vi "Send signal mode.vi"() -> ()   [LabVIEW 2020]
uses:
  <vilib>/xnet/xnet.llb/XNET Write (Signal Single-point).vi
  <vilib>/xnet/xnet.llb/XNET Create Session (Signal Output Single-point).vi
panel:
  out "校验成功":bool=TRUE
  in  "Close":bool
  in  "CAN1_interface":refnum<k21>="CAN1"
  in  "CAN1":refnum<k21>[](array[refnum])=["Vehicle_speed\nSA2HG", "VehicleSpeed_Status\nSA2HG", "ESP1_MSG_Counter\nSA2HG", "ESP1_Checksum\nSA2HG"]
  in  "CAN1_Write":bool
  in  "CAN1_commd":dbl[](array[numeric])=[0.0, 0.0, 0.0, 0.0] caption="data"
  in  "CAN2_Stop":bool
  in  "CAN1_Stop":bool
  in  "CAN2_Write":bool
  in  "CAN2_commd":dbl[](array[numeric])=[0.0, 0.0, 0.0, 0.0, 0.0] caption="data"
  in  "CAN_Interface":refnum<k21>="CAN1"
  in  "CAN2":refnum<k21>[](array[refnum])=["READY\nSA2HG"]
  # "发送车速信号，时间间隔20ms"
  # "发送Ready信号，时间间隔为100ms"
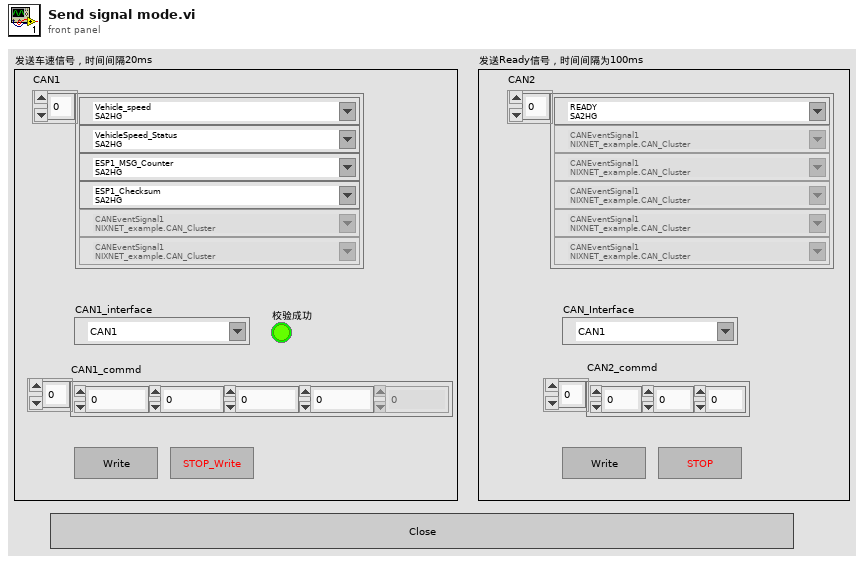
[diagram p1: front panel]
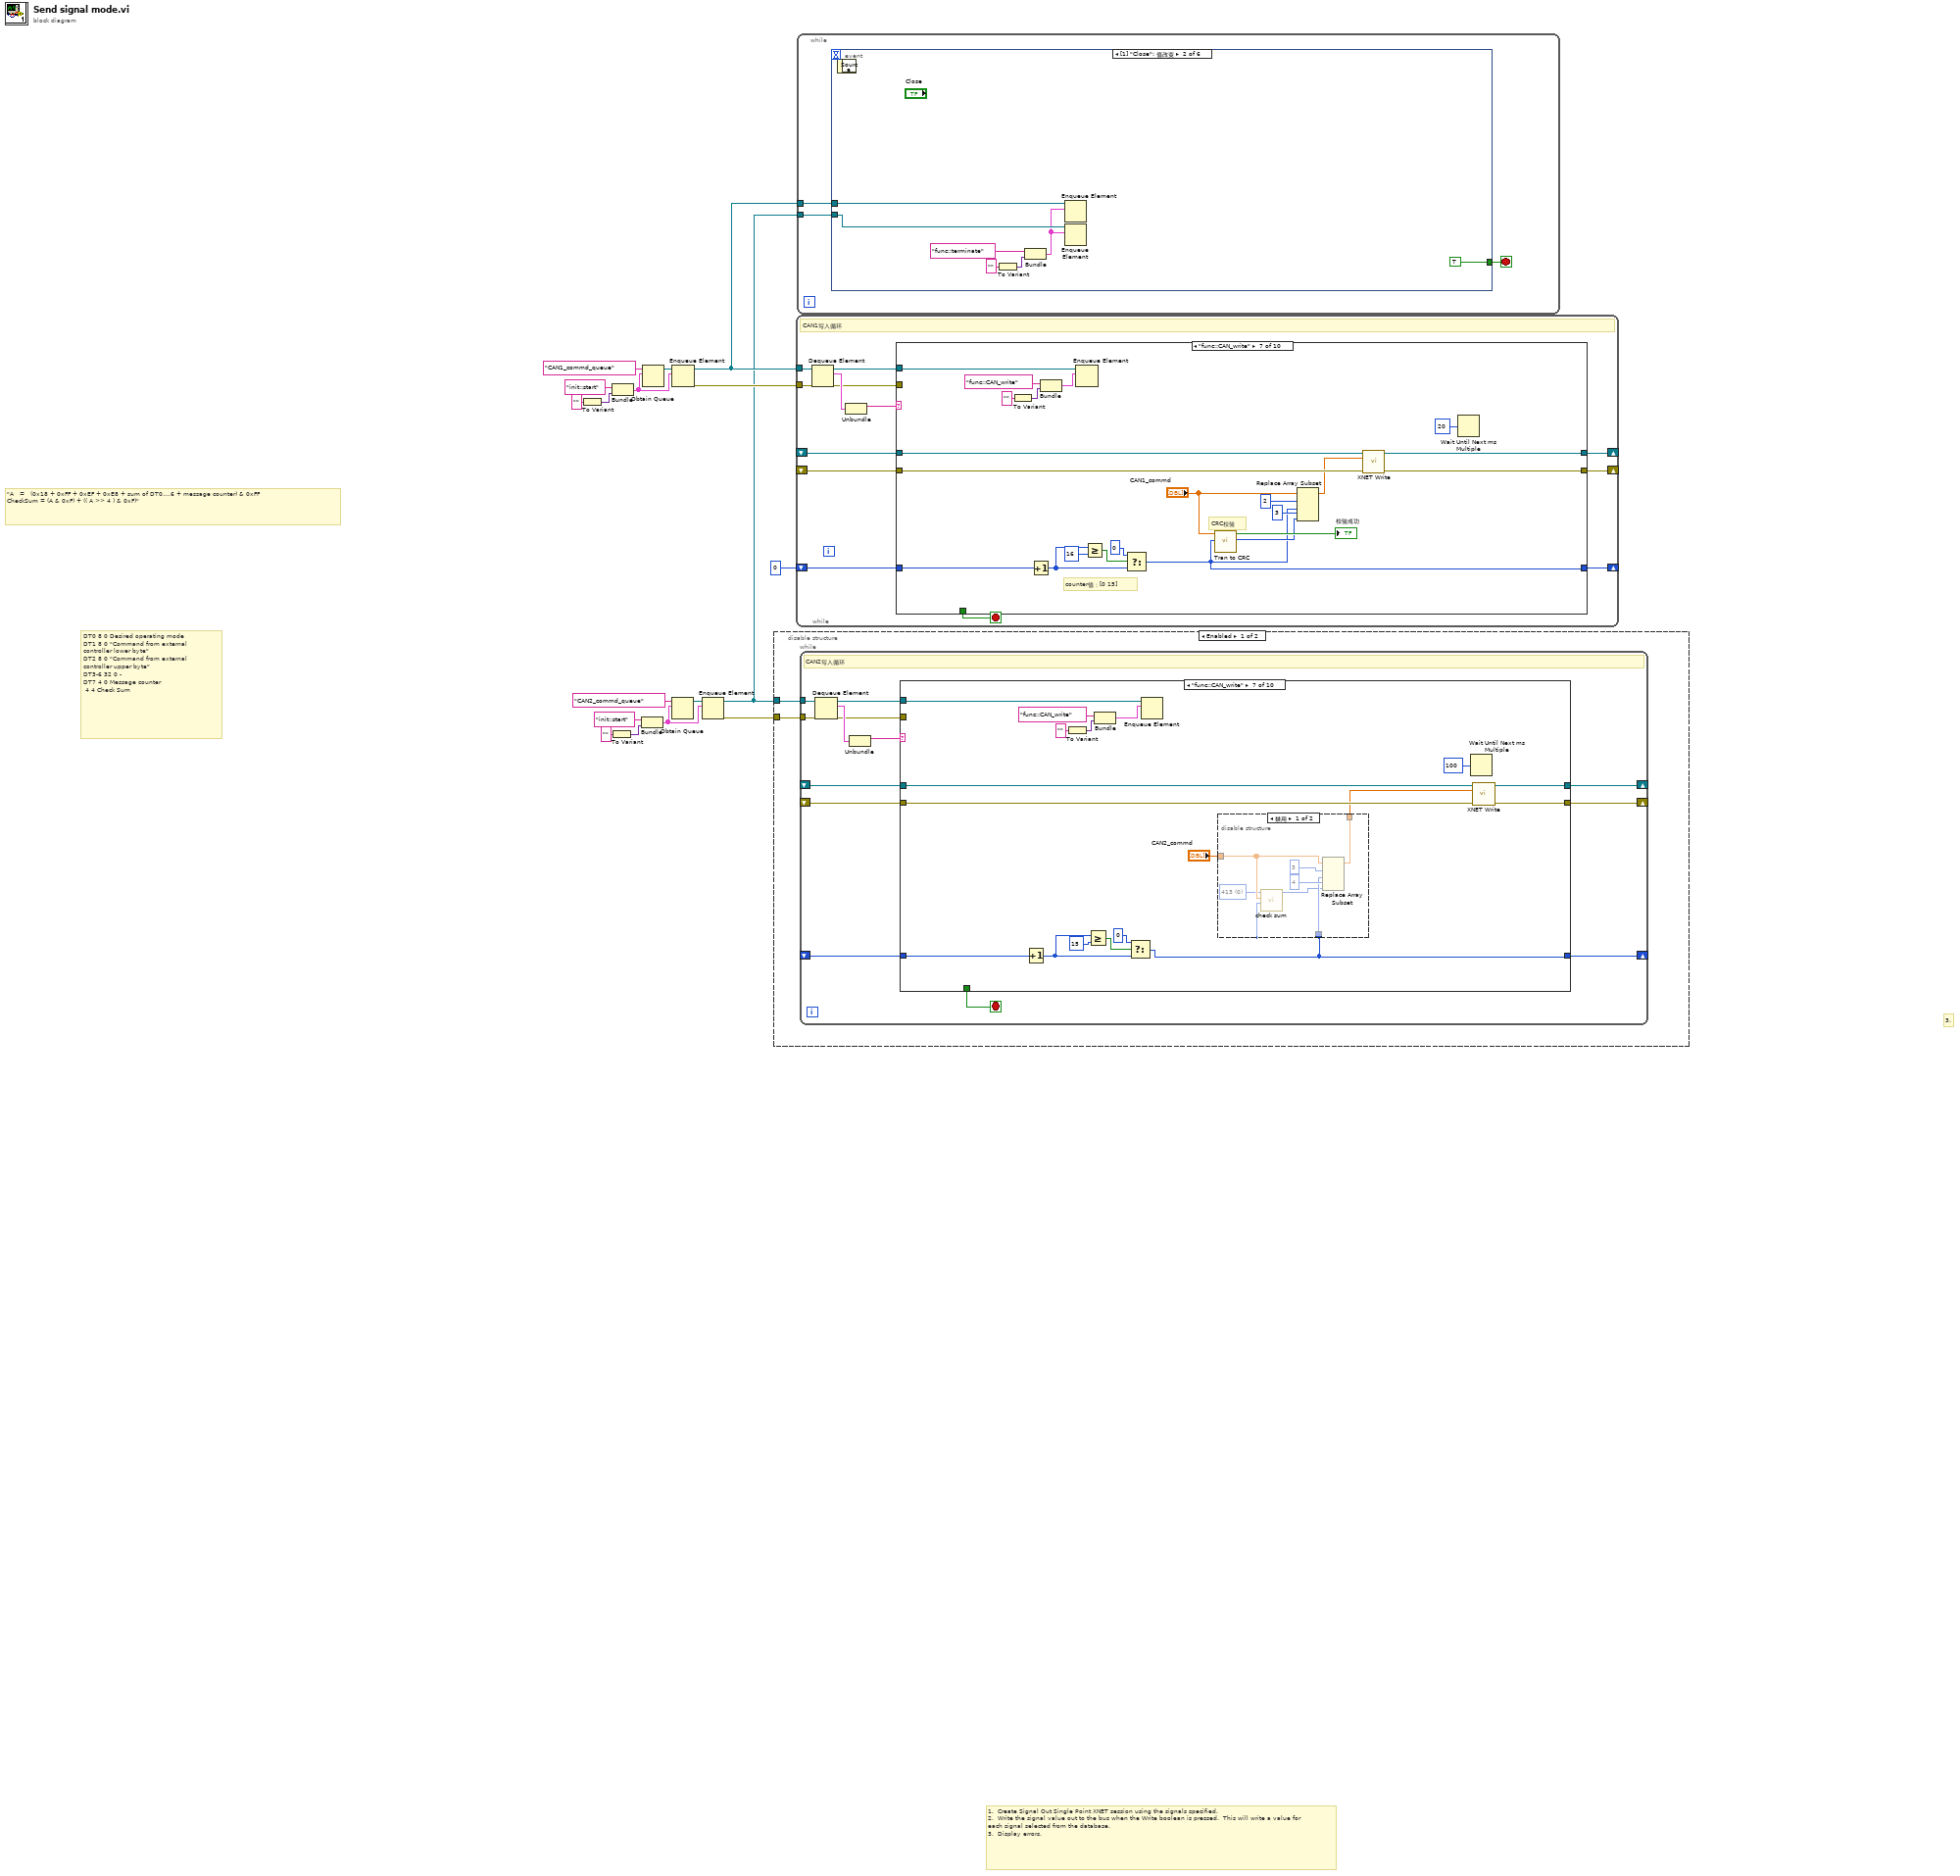
[diagram p0: block diagram]
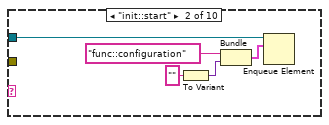
[diagram p3: hidden frame]
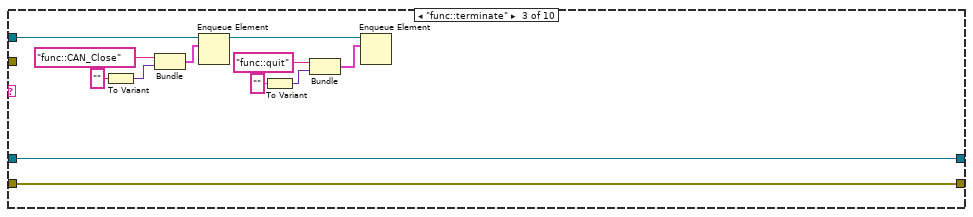
[diagram p4: hidden frame]
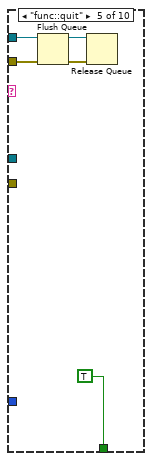
[diagram p6: hidden frame]
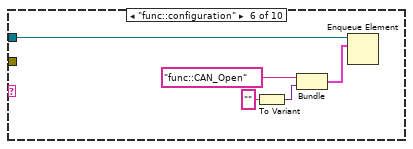
[diagram p7: hidden frame]
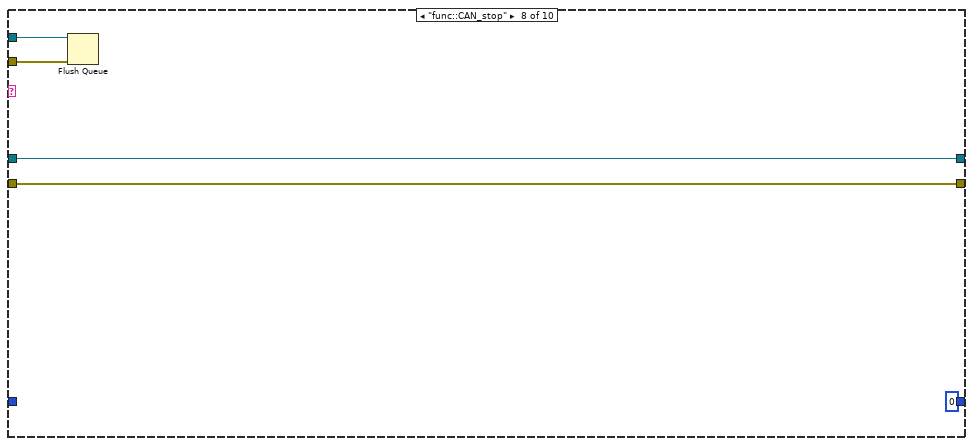
[diagram p9: hidden frame]
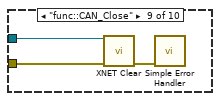
[diagram p10: hidden frame]
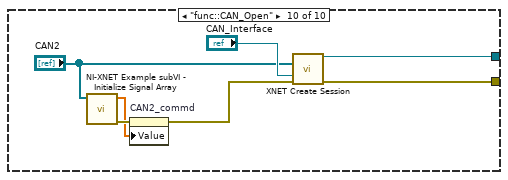
[diagram p11: hidden frame]
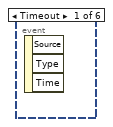
[diagram p13: hidden frame]
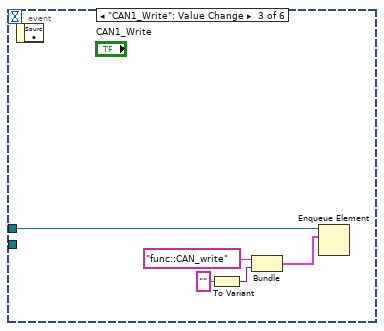
[diagram p14: hidden frame]
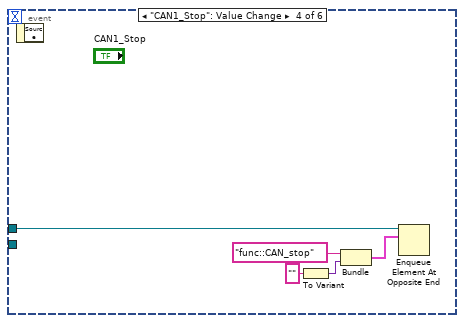
[diagram p15: hidden frame]
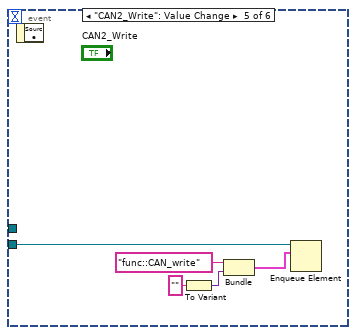
[diagram p16: hidden frame]
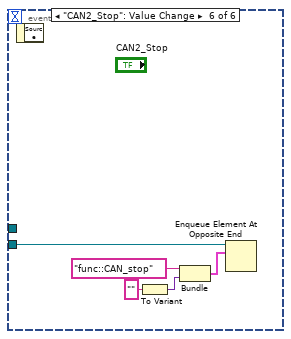
[diagram p17: hidden frame]
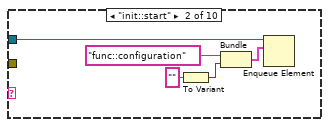
[diagram p19: hidden frame]
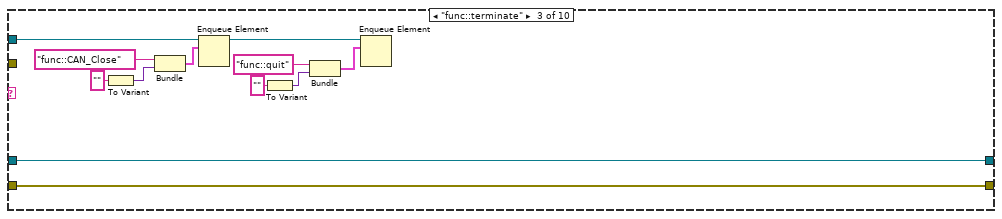
[diagram p20: hidden frame]
diagram:
  # "DT0\t8\t0\tDesired operating mode\nDT1\t8\t0\t\"Command from external\ncontroller lower byte\"\nDT2\t8\t0\t\"Command from external\ncontroller upper byte\"\nDT3-6\t32\t0\t-\nDT7\t4\t0\tMessage counter\n\t4\t4\tCheck Sum"
  # "\"A　=　(0x18 + 0xFF + 0xEF + 0xE8 + sum of DT0….6 + message counter) & 0xFF\nCheckSum = (A & 0xF) + (( A >> 4 ) & 0xF)\""
  # "3."
  # "1.  Create Signal Out Single Point XNET session using the signals specified.  \n2.  Write the signal value out to the bus when the Write boolean is pressed.  This will write a value for each signal selected from the database.\n3.  Display errors."
  n1 = To Variant(anything="") -> (Variant=w15:variant)
  n2 = To Variant(anything="") -> (Variant=w4:variant)
  n3 = Bundle("init::start", "Variant"=w15) -> (w13:cluster{string, "Variant":variant})  [unwired: 1 in]
  n4 = Bundle("init::start", "Variant"=w4) -> (w6:cluster{string, "Variant":variant})  [unwired: 1 in]
  n5 = Obtain Queue(name (unnamed)="CAN1_commd_queue", element data type=w13) -> (queue out=w14:refnum<queue>)  [unwired: 3 in, 2 out]
  n6 = Obtain Queue(name (unnamed)="CAN2_commd_queue", element data type=w6) -> (queue out=w5:refnum<queue>)  [unwired: 3 in, 2 out]
  n7 = Enqueue Element(queue=w14, element=w13) -> (queue out=w10:refnum<queue>, error out=w9:errorcluster)  [unwired: 2 in, 1 out]
  n8 = Enqueue Element(queue=w5, element=w6) -> (queue out=w8:refnum<queue>, error out=w1:errorcluster)  [unwired: 2 in, 1 out]
  n9 = disable-structure shown="Enabled" {
    disable-tunnel: w8 -> [w19 _]
    disable-tunnel: w1 -> [w18 _]
    frame Enabled {
      n10 = while {
        tunnel: w19 -> [w31]
        tunnel: w18 -> [w28]
        shift-right: [w25] -> _
        shift-left: _ -> [w23]
        shift-right: [w24] -> _
        shift-left: _ -> [w22]
        shift-right: [w20] -> _
        shift-left: _ -> [w21]
        stop <- w26 stop-if-true
        # "CAN2写入循环"
        n11 = Dequeue Element(queue=w31, error in (no error)=w28) -> (queue out=w29:refnum<queue>, element=w32:cluster{string, "Variant":variant}, error out=w27:errorcluster)  [unwired: 1 in, 1 out]
        n12 = Unbundle(w32) -> (w30:string)  [unwired: 1 out]
        n13 = case shown="\"func::CAN_write\"" w30 {
          tunnel: w29 -> [_ w34 w40 _ w52 w55 w64 w88 _ _]
          tunnel: w27 -> [_ _ _ _ w51 _ _ w87 _ _]
          tunnel: [_ _ _ _ TRUE _ _ _ _ _] -> w26
          tunnel: [_ _ w39 _ _ _ w77 w90 _ w95] -> w25
          tunnel: [_ _ w38 _ _ _ w76 w89 _ w94] -> w24
          tunnel: w23 -> [_ _ w39 _ _ _ w75 w90 w92 _]
          tunnel: w22 -> [_ _ w38 _ _ _ w74 w89 w91 _]
          tunnel: w21 -> [_ _ _ _ _ _ w69 _ _ _]
          tunnel: [_ _ _ _ _ _ w61 0 _ _] -> w20
          frame Default {
          }
          frame "init::start" {
            n14 = To Variant(anything="") -> (Variant=w36:variant)
            n15 = Bundle("func::configuration", "Variant"=w36) -> (w35:cluster{string, "Variant":variant})  [unwired: 1 in]
            n16 = Enqueue Element(queue=w34, element=w35) -> ()  [unwired: 2 in, 3 out]
          }
          frame "func::terminate" {
            n17 = To Variant(anything="") -> (Variant=w48:variant)
            n18 = Bundle("func::CAN_Close", "Variant"=w48) -> (w46:cluster{string, "Variant":variant})  [unwired: 1 in]
            n19 = Enqueue Element(queue=w40, element=w46) -> (queue out=w41:refnum<queue>)  [unwired: 2 in, 2 out]
            n20 = To Variant(anything="") -> (Variant=w44:variant)
            n21 = Bundle("func::quit", "Variant"=w44) -> (w42:cluster{string, "Variant":variant})  [unwired: 1 in]
            n22 = Enqueue Element(queue=w41, element=w42) -> ()  [unwired: 2 in, 3 out]
          }
          frame "func::close" {
          }
          frame "func::quit" {
            n23 = Flush Queue(queue=w52, error in (no error)=w51) -> (queue out=w54:refnum<queue>, error out=w53:errorcluster)  [unwired: 1 out]
            n24 = Release Queue(queue=w54, error in (no error)=w53) -> ()  [unwired: 1 in, 3 out]
          }
          frame "func::configuration" {
            n25 = To Variant(anything="") -> (Variant=w59:variant)
            n26 = Bundle("func::CAN_Open", "Variant"=w59) -> (w58:cluster{string, "Variant":variant})  [unwired: 1 in]
            n27 = Enqueue Element(queue=w55, element=w58) -> ()  [unwired: 2 in, 3 out]
          }
          frame "func::CAN_write" {
            n28 = Increment(x=w69) -> (x+1=w73:i32)
            n29 = To Variant(anything="") -> (Variant=w67:variant)
            n30 = Greater Or Equal?(x=w73, y=15) -> (x >= y?=w70:bool)
            n31 = Bundle("func::CAN_write", "Variant"=w67) -> (w66:cluster{string, "Variant":variant})  [unwired: 1 in]
            n32 = Select(t=0, s=w70, f=w73) -> (s? t:f=w61:i32)
            n33 = Enqueue Element(queue=w64, element=w66) -> ()  [unwired: 2 in, 3 out]
            n34 = disable-structure shown="禁用" {
              disable-tunnel: "CAN2_commd" -> [w82 w85]
              disable-tunnel: w61 -> [w81 _]
              disable-tunnel: [w79 w85] -> w60
              frame Disabled {
                w78 = u16 0 items=["413", "18FFEFE8"] ("ID")
                n35 = call "check sum.vi"("counter up"=w81, "CAN_commd"=w82, "ID"=w78) -> ("check sum"=w80:u32)  [unwired: 8 in]
                n36 = Replace Array Subset(array=w82, new element #1=w81, index #1=3 ("索引"), new element #2=w80, index #2=4 ("索引")) -> (w79:dbl[])
              }
              frame Enabled {
              }
            }
            n37 = Wait Until Next ms Multiple(millisecond multiple=u32 100 ("milliseconds to wait")) -> ()  [unwired: 1 out]
            n38 = call-poly <vilib>:"XNET Write.vi"("session in"=w75, "data"=w60, "error in (no error)"=w74) -> ("session out"=w77:refnum<k21>, "error out"=w76:errorcluster)  [unwired: 11 out]
          }
          frame "func::CAN_stop" {
            n39 = Flush Queue(queue=w88, error in (no error)=w87) -> ()  [unwired: 3 out]
          }
          frame "func::CAN_Close" {
            n40 = call <vilib>:"XNET Clear.vi"("session in"=w92, "error in (no error)"=w91) -> ("error out"=w93:errorcluster)  [unwired: 13 in]
            n41 = call <vilib>:"Simple Error Handler.vi"("error in (no error)"=w93) -> ()  [unwired: 4 in, 5 out]
          }
          frame "func::CAN_Open" {
            n42 = call "NI-XNET Example subVI - Initialize Signal Array.vi"("signal list"="CAN2") -> ("error out"=w97:errorcluster, "Default Values"=w96:dbl[])  [unwired: 1 in, 6 out]
            n43 = property on="CAN2_commd" class="Arr (严格)"(error in=w97, "Value"=w96) -> (error out=w98:errorcluster)  [unwired: 1 in, 1 out]
            n44 = call-poly <vilib>:"XNET Create Session.vi"("signal list"="CAN2", "interface"="CAN_Interface", "error in (no error)"=w98) -> ("session out"=w95:refnum<k21>, "error out"=w94:errorcluster)  [unwired: 11 out]
          }
        }
      }
    }
    frame Disabled {
    }
  }
  n45 = while {
    tunnel: w10 -> [w112]
    tunnel: w9 -> [w109]
    shift-right: [w106] -> _
    shift-left: _ -> [w104]
    shift-right: [w105] -> _
    shift-left: _ -> [w103]
    shift-right: [w101] -> _
    shift-left: 0 -> [w102]
    stop <- w107 stop-if-true
    # "CAN1写入循环"
    n46 = Dequeue Element(queue=w112, error in (no error)=w109) -> (queue out=w110:refnum<queue>, element=w113:cluster{string, "Variant":variant}, error out=w108:errorcluster)  [unwired: 1 in, 1 out]
    n47 = Unbundle(w113) -> (w111:string)  [unwired: 1 out]
    n48 = case shown="\"func::CAN_write\"" w111 {
      tunnel: w110 -> [_ w115 w121 _ w133 w136 w148 w165 _ _]
      tunnel: w108 -> [_ _ _ _ w132 _ _ w164 _ _]
      tunnel: [_ _ _ _ TRUE _ _ _ _ _] -> w107
      tunnel: [_ _ w120 _ _ _ w160 w167 _ w172] -> w106
      tunnel: [_ _ w119 _ _ _ w159 w166 _ w171] -> w105
      tunnel: w104 -> [_ _ w120 _ _ _ w158 w167 w169 _]
      tunnel: w103 -> [_ _ w119 _ _ _ w157 w166 w168 _]
      tunnel: w102 -> [_ _ _ _ _ _ w146 _ _ _]
      tunnel: [_ _ _ _ _ _ w141 0 _ _] -> w101
      frame Default {
      }
      frame "init::start" {
        n49 = To Variant(anything="") -> (Variant=w117:variant)
        n50 = Bundle("func::configuration", "Variant"=w117) -> (w116:cluster{string, "Variant":variant})  [unwired: 1 in]
        n51 = Enqueue Element(queue=w115, element=w116) -> ()  [unwired: 2 in, 3 out]
      }
      frame "func::terminate" {
        n52 = To Variant(anything="") -> (Variant=w129:variant)
        n53 = Bundle("func::CAN_Close", "Variant"=w129) -> (w127:cluster{string, "Variant":variant})  [unwired: 1 in]
        n54 = Enqueue Element(queue=w121, element=w127) -> (queue out=w122:refnum<queue>)  [unwired: 2 in, 2 out]
        n55 = To Variant(anything="") -> (Variant=w125:variant)
        n56 = Bundle("func::quit", "Variant"=w125) -> (w123:cluster{string, "Variant":variant})  [unwired: 1 in]
        n57 = Enqueue Element(queue=w122, element=w123) -> ()  [unwired: 2 in, 3 out]
      }
      frame "func::close" {
      }
      frame "func::quit" {
        n58 = Flush Queue(queue=w133, error in (no error)=w132) -> (queue out=w135:refnum<queue>, error out=w134:errorcluster)  [unwired: 1 out]
        n59 = Release Queue(queue=w135, error in (no error)=w134) -> ()  [unwired: 1 in, 3 out]
      }
      frame "func::configuration" {
        n60 = To Variant(anything="") -> (Variant=w140:variant)
        n61 = Bundle("func::CAN_Open", "Variant"=w140) -> (w139:cluster{string, "Variant":variant})  [unwired: 1 in]
        n62 = Enqueue Element(queue=w136, element=w139) -> ()  [unwired: 2 in, 3 out]
      }
      frame "func::CAN_write" {
        # "CRC校验"
        # "counter值：[0 15]"
        n63 = To Variant(anything="") -> (Variant=w151:variant)
        n64 = Increment(x=w146) -> (x+1=w156:i32)
        n65 = Bundle("func::CAN_write", "Variant"=w151) -> (w150:cluster{string, "Variant":variant})  [unwired: 1 in]
        n66 = Enqueue Element(queue=w148, element=w150) -> ()  [unwired: 2 in, 3 out]
        n67 = Greater Or Equal?(x=w156, y=16) -> (x >= y?=w153:bool)
        n68 = Select(t=0, s=w153, f=w156) -> (s? t:f=w141:i32)
        n69 = call "Tran to CRC.vi"("Counter"=w141, "CAN_commd"="CAN1_commd") -> ("校验值"=w143:u64, "校验成功"=→"校验成功":bool)  [unwired: 5 in, 1 out]
        n70 = Replace Array Subset(array="CAN1_commd", new element #1=w141, index #1=2 ("index"), new element #2=w143, index #2=3 ("index")) -> (w145:dbl[])
        n71 = call-poly <vilib>:"XNET Write.vi"("session in"=w158, "data"=w145, "error in (no error)"=w157) -> ("session out"=w160:refnum<k21>, "error out"=w159:errorcluster)  [unwired: 11 out]
        n72 = Wait Until Next ms Multiple(millisecond multiple=u32 20 ("milliseconds to wait")) -> ()  [unwired: 1 out]
      }
      frame "func::CAN_stop" {
        n73 = Flush Queue(queue=w165, error in (no error)=w164) -> ()  [unwired: 3 out]
      }
      frame "func::CAN_Close" {
        n74 = call <vilib>:"XNET Clear.vi"("session in"=w169, "error in (no error)"=w168) -> ("error out"=w170:errorcluster)  [unwired: 13 in]
        n75 = call <vilib>:"Simple Error Handler.vi"("error in (no error)"=w170) -> ()  [unwired: 4 in, 5 out]
      }
      frame "func::CAN_Open" {
        n76 = call "NI-XNET Example subVI - Initialize Signal Array.vi"("signal list"="CAN1") -> ("error out"=w174:errorcluster, "Default Values"=w175:dbl[])  [unwired: 1 in, 6 out]
        n77 = property on="CAN1_commd" class="Arr (严格)"(error in=w174, "Value"=w175) -> (error out=w173:errorcluster)  [unwired: 1 in, 1 out]
        n78 = call-poly <vilib>:"XNET Create Session.vi"("signal list"="CAN1", "interface"="CAN1_interface", "error in (no error)"=w173) -> ("session out"=w172:refnum<k21>, "error out"=w171:errorcluster)  [unwired: 11 out]
      }
    }
  }
  n79 = while {
    tunnel: w10 -> [w180]
    tunnel: w8 -> [w179]
    stop <- w178 stop-if-true
    n80 = event shown="[1] \"Close\": 值改变" {
      selector: _ -> [_ _ _ _ _ _]
      dyn-events: _ -> [_ _ _ _ _ _]
      timeout: _ -> [_ _ _ _ _ _]
      tunnel: w180 -> [_ w184 w188 w194 _ _]
      tunnel: w179 -> [_ w183 _ _ w198 w204]
      tunnel: [_ TRUE _ _ _ _] -> w178
      event Timeout {
        n81 = event-data() -> ()  [unwired: 1 in, 3 out]
      }
      event "Close": Value Change {
        n82 = event-data() -> ()  [unwired: 1 in, 1 out]
        n83 = To Variant(anything="") -> (Variant=w186:variant)
        n84 = Bundle("func::terminate", "Variant"=w186) -> (w182:cluster{string, "Variant":variant})  [unwired: 1 in]
        n85 = Enqueue Element(queue=w184, element=w182) -> ()  [unwired: 2 in, 3 out]
        n86 = Enqueue Element(queue=w183, element=w182) -> ()  [unwired: 2 in, 3 out]
      }
      event "CAN1_Write": Value Change {
        n87 = event-data() -> ()  [unwired: 1 in, 1 out]
        n88 = To Variant(anything="") -> (Variant=w190:variant)
        n89 = Bundle("func::CAN_write", "Variant"=w190) -> (w191:cluster{string, "Variant":variant})  [unwired: 1 in]
        n90 = Enqueue Element(queue=w188, element=w191) -> ()  [unwired: 2 in, 3 out]
      }
      event "CAN1_Stop": Value Change {
        n91 = event-data() -> ()  [unwired: 1 in, 1 out]
        n92 = To Variant(anything="") -> (Variant=w196:variant)
        n93 = Bundle("func::CAN_stop", "Variant"=w196) -> (w193:cluster{string, "Variant":variant})  [unwired: 1 in]
        n94 = Enqueue Element At Opposite End(queue=w194, element=w193) -> ()  [unwired: 2 in, 3 out]
      }
      event "CAN2_Write": Value Change {
        n95 = event-data() -> ()  [unwired: 1 in, 1 out]
        n96 = To Variant(anything="") -> (Variant=w201:variant)
        n97 = Bundle("func::CAN_write", "Variant"=w201) -> (w202:cluster{string, "Variant":variant})  [unwired: 1 in]
        n98 = Enqueue Element(queue=w198, element=w202) -> ()  [unwired: 2 in, 3 out]
      }
      event "CAN2_Stop": Value Change {
        n99 = event-data() -> ()  [unwired: 1 in, 1 out]
        n100 = To Variant(anything="") -> (Variant=w207:variant)
        n101 = Bundle("func::CAN_stop", "Variant"=w207) -> (w203:cluster{string, "Variant":variant})  [unwired: 1 in]
        n102 = Enqueue Element At Opposite End(queue=w204, element=w203) -> ()  [unwired: 2 in, 3 out]
      }
    }
  }
